vi "Begin.vi"() -> (0 "error out":errorcluster)   [LabVIEW 2013]
doc: "Called before other user functions, this VI is expected to open initial I/O refnums, load in file data, and do all program initialization. Notice that the <B>error out</B> terminal is simply used for data flow. Wiring it to other structures or subVIs ensures that this VI runs first."
uses:
  <vilib>/Rock Robotics/WPI/SafetyOutput/WPI_SafetyOutputConfigMenu.ctl
  <vilib>/Rock Robotics/WPI/DriverStation/WPI_DriverStationRobotMode2.ctl
  <vilib>/Rock Robotics/WPI/Joystick/WPI_JoystickDeviceEnum.ctl
  <vilib>/Rock Robotics/SystemInterfaces/DIO/FPGA_DIOPWMChannel.ctl
  <vilib>/Rock Robotics/SystemInterfaces/DIO/FPGA_DIORelayChannel.ctl
  <vilib>/Rock Robotics/WPI/Solenoid/WPI_SolenoidChannel.ctl
  <vilib>/Rock Robotics/SystemInterfaces/DIO/FPGA_DIOChannel.ctl
  <vilib>/Rock Robotics/SystemInterfaces/Typedef/FPGA_TypedefSolenoidModule.ctl
  <vilib>/Rock Robotics/WPI/Solenoid/WPI_SolenoidValue.ctl
  <vilib>/Rock Robotics/SystemInterfaces/Typedef/FPGA_TypedefAnalogModule.ctl
  <vilib>/Rock Robotics/SystemInterfaces/AI/FPGA_AIChannel.ctl
  <vilib>/Rock Robotics/SystemInterfaces/Typedef/FPGA_TypedefDigitalModule.ctl
  Robot Global Data.vi
  <vilib>/Rock Robotics/WPI/RobotDrive/WPI_RobotDriveOpen4MotorWithJaguar.vi
  <vilib>/Rock Robotics/WPI/MotorControl/WPI_MotorControlOpen Jaguar.vi
  <vilib>/Rock Robotics/WPI/Solenoid/WPI_SolenoidOpenDouble.vi
  <vilib>/Rock Robotics/WPI/Solenoid/WPI_SolenoidSetEnum.vi
  <vilib>/Rock Robotics/WPI/MotorControl/WPI_MotorControlOpen Victor.vi
  <vilib>/Rock Robotics/WPI/Compressor/WPI_CompressorGetSetRefNum.vi
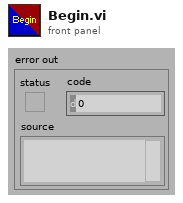
[diagram p1: front panel]
types:
  T1 = typedef "FPGA_TypedefDigitalModule.ctl" = enum16{"Digital Module 1", "Digital Module 2"}
  T2 = typedef "FPGA_DIORelayChannel.ctl" = enum8{"Relay 1", "Relay 2", "Relay 3", "Relay 4", "Relay 5", "Relay 6", "Relay 7", "Relay 8", "Invalid"}
  T3 = typedef "FPGA_AIChannel.ctl" = enum8{"AI 1", "AI 2", "AI 3", "AI 4", "AI 5", "AI 6", "AI 7", "AI 8", "Invalid"}
  T4 = typedef "FPGA_TypedefAnalogModule.ctl" = enum16{"Analog Module 1", "Analog Module 2"}
  T5 = typedef "WPI_SolenoidValue.ctl" = enum16{"Off", "On", "Forward", "Reverse"}
  T6 = typedef "WPI_SolenoidChannel.ctl" = enum8{"Solenoid 1", "Solenoid 2", "Solenoid 3", "Solenoid 4", "Solenoid 5", "Solenoid 6", "Solenoid 7", "Solenoid 8", "Invalid"}
  T7 = typedef "FPGA_TypedefSolenoidModule.ctl" = enum16{"Solenoid Module 1", "Solenoid Module 2"}
  T8 = typedef "FPGA_DIOPWMChannel.ctl" = enum8{"PWM 1", "PWM 2", "PWM 3", "PWM 4", "PWM 5", "PWM 6", "PWM 7", "PWM 8", "PWM 9", "PWM 10", "Invalid"}
  T9 = typedef "FPGA_DIOChannel.ctl" = enum8{"DIO 1", "DIO 2", "DIO 3", "DIO 4", "DIO 5", "DIO 6", "DIO 7", "DIO 8", "DIO 9", "DIO 10", "DIO 11", "DIO 12", "DIO 13", "DIO 14", "Invalid"}
  T10 = typedef "WPI_JoystickDeviceEnum.ctl" = enum16{"USB 1", "USB 2", "USB 3", "USB 4", "Kinect 1", "Kinect 2"}
  T11 = typedef "WPI_DriverStationRobotMode2.ctl" = enum16{"Autonomous Disabled", "Autonomous Enabled", "Teleop Disabled", "Teleop Enabled", "Timeout", "Finish", "Test Disabled", "Test Enabled"}
  T12 = typedef "WPI_SafetyOutputConfigMenu.ctl" = enum16{"Enable", "Disable"}
  T13 = typedef "WPI_MotorControlDeviceRef.ctl" = cluster{"DeviceStatus":errorcluster, "Type":enum16{"PWM", "CAN"}, "PWM":cluster{"Digital Module":T1, "PWM Channel":T8, "DeadBand":T14}, "CAN":cluster{"Device Number":u8, "Control Mode":T15, "Semaphore":T16, "Max Vout":dbl}, "Invert":bool, "TransformRef":T17, "InvTransformRef":T17}
  T14 = typedef "WPI_PWMDeadband.ctl" = cluster{"Name":string, "maxPositivePwm":i32, "minPositivePwm":i32, "centerPwm":i32, "maxNegativePwm":i32, "minNegativePwm":i32, "angularRange":u16}
  T15 = typedef "WPI_CANJaguar_ControlMode.ctl" = enum8{"Percent VBus", "Current", "Speed", "Position", "Voltage"}
  T16 = typedef "Semaphore RefNum" = refnum<k1>
  T17 = typedef "WPI_PWMTransform_ConPane.ctl" = refnum<vi>
  T18 = typedef "WPI_JoystickDevRef.ctl" = cluster{"Device":T10}
  T19 = typedef "WPI_RobotDriveDevRef.ctl" = cluster{"DevStatus":errorcluster, "Motors[]":T13[], "Square Inputs":bool, "Max Output":dbl, "Isochronous":bool}
  T20 = typedef "WPI_SolenoidDevRef.ctl" = cluster{"DevStatus":errorcluster, "Solenoid Module":T7, "Forward Solenoid Channel":T6, "Reverse Solenoid Channel":T6}
  T21 = typedef "WPI_RelayDevRef.ctl" = cluster{"DevStatus":errorcluster, "Relay Channel":T2, "Digital Module":T1, "Relay Direction":T22}
  T22 = typedef "WPI_RelayDirection.ctl" = enum16{"Both directions", "Forward only", "Reverse only"}
  T23 = typedef "WPI_CompressorDevRef.ctl" = cluster{"DevStatus":errorcluster, "DigitalInputDevRef":T24, "RelayDevRef":T21}
  T24 = typedef "WPI_DigitalInputDevRef.ctl" = cluster{"DevStatus":errorcluster, "DIO Channel":T9, "Digital Module":T1}
  T25 = typedef "WPI_AnalogChannelDevRef.ctl" = cluster{"DevStatus":errorcluster, "Analog Module":T4, "Analog Channel":T3}
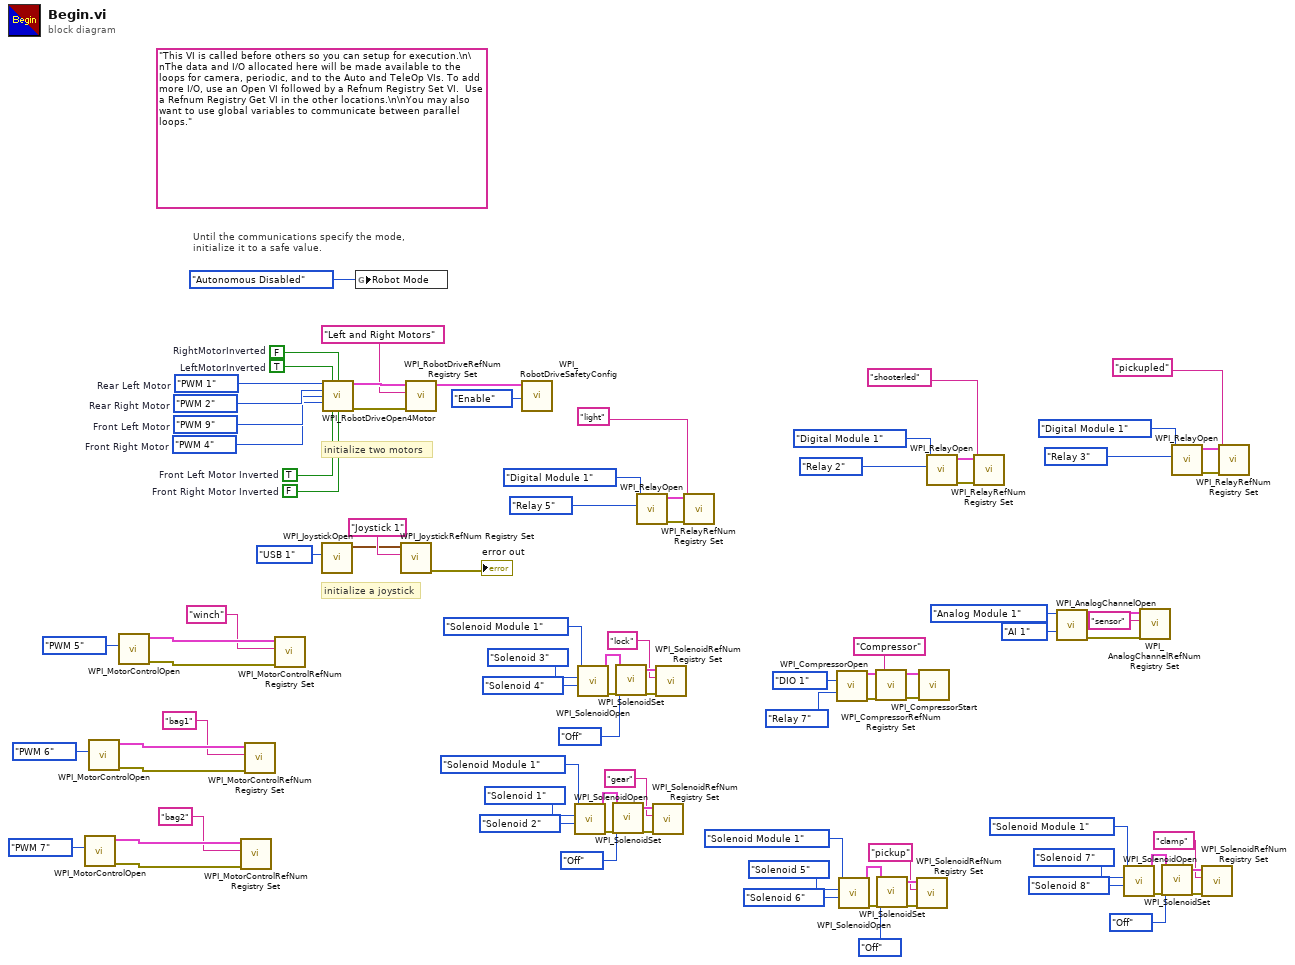
[diagram p0: block diagram]
diagram:
  w76 = FALSE  # Front Right Motor Inverted
  w77 = TRUE  # Front Left Motor Inverted
  w78 = FPGA_DIOPWMChannel."PWM 4"  # Front Right Motor
  w79 = FPGA_DIOPWMChannel."PWM 9"  # Front Left Motor
  w80 = FPGA_DIOPWMChannel."PWM 2"  # Rear Right Motor
  w81 = FPGA_DIOPWMChannel."PWM 1"  # Rear Left Motor
  (unwired) "This VI is called before others so you can setup for execution.\n\nThe data and I/O allocated here will be made available to the loops for camera, periodic, and to the Auto and TeleOp VIs. To add more I/O, use an Open VI followed by a Refnum Registry Set VI.  Use a Refnum Registry Get VI in the other locations.\n\nYou may also want to use global variables to communicate between parallel loops."
  w92 = TRUE  # LeftMotorInverted
  w93 = FALSE  # RightMotorInverted
  # "initialize a joystick"
  # "Until the communications specify the mode,\ninitialize it to a safe value."
  # "initialize two motors"
  n1 = call-poly <vilib>:"WPI_MotorControlOpen.vi"("PWM Channel"=FPGA_DIOPWMChannel."PWM 7") -> ("error out"=w32:errorcluster, "MotorControlDeviceRef"=w31:T13)  [unwired: 9 in]
  n2 = call-poly <vilib>:"WPI_MotorControlOpen.vi"("PWM Channel"=FPGA_DIOPWMChannel."PWM 6") -> ("error out"=w43:errorcluster, "MotorControlDeviceRef"=w42:T13)  [unwired: 9 in]
  n3 = call-poly <vilib>:"WPI_MotorControlOpen.vi"("PWM Channel"=FPGA_DIOPWMChannel."PWM 5") -> ("error out"=w69:errorcluster, "MotorControlDeviceRef"=w68:T13)  [unwired: 9 in]
  n4 = call <vilib>:"WPI_MotorControlRefNum Registry Set.vi"("error in (no error)"=w32, "refnum name"="bag2", "MotorControlDevRef"=w31) -> ()  [unwired: 7 in, 2 out]
  n5 = call <vilib>:"WPI_MotorControlRefNum Registry Set.vi"("error in (no error)"=w43, "refnum name"="bag1", "MotorControlDevRef"=w42) -> ()  [unwired: 7 in, 2 out]
  n6 = call <vilib>:"WPI_MotorControlRefNum Registry Set.vi"("error in (no error)"=w69, "refnum name"="winch", "MotorControlDevRef"=w68) -> ()  [unwired: 7 in, 2 out]
  n7 = call <vilib>:"WPI_JoystickOpen.vi"("JoystickDevice"=WPI_JoystickDeviceEnum."USB 1") -> ("JoystickDevRef"=w84:T18)  [unwired: 10 in]
  n8 = call-poly <vilib>:"WPI_RobotDriveOpen4Motor.vi"("Rear Left Motor"=w81, "Rear Left Motor Inverted"=w92, "Rear Right Motor Inverted"=w93, "Rear Right Motor"=w80, "Front Left Motor"=w79, "Front Right Motor"=w78, "Front Left Motor Inverted"=w77, "Front Right Motor Inverted"=w76) -> ("RobotDriveDevRef"=w91:T19, "error out"=w89:errorcluster)  [unwired: 6 in]
  n9 = global write "Robot Global Data.vi" "Robot Mode"(WPI_DriverStationRobotMode2."Autonomous Disabled" ("Robot Mode")) -> ()
  n10 = call <vilib>:"WPI_JoystickRefNum Registry Set.vi"("refnum name"="Joystick 1", "JoystickDevRef"=w84) -> ("error out"=→"error out":errorcluster)  [unwired: 8 in, 1 out]
  n11 = call <vilib>:"WPI_RobotDriveRefNum Registry Set.vi"("error in (no error)"=w89, "refnum name"="Left and Right Motors", "RobotDriveDevRef"=w91) -> ("RobotDriveDevRef"=w88:T19)  [unwired: 8 out]
  n12 = call <vilib>:"WPI_RobotDriveSafetyConfig.vi"("mode"=WPI_SafetyOutputConfigMenu."Enable", "RobotDriveDevRef"=w88) -> ()  [unwired: 8 in, 2 out]
  n13 = call-poly <vilib>:"WPI_SolenoidOpen.vi"("Reverse Solenoid Channel"=WPI_SolenoidChannel."Solenoid 2", "Forward Solenoid Channel"=WPI_SolenoidChannel."Solenoid 1" ("Solenoid Channel"), "Solenoid Module (Module 1)"=FPGA_TypedefSolenoidModule."Solenoid Module 1") -> ("error out"=w54:errorcluster, "SolenoidDevRef"=w53:T20)  [unwired: 7 in]
  n14 = call-poly <vilib>:"WPI_SolenoidOpen.vi"("Reverse Solenoid Channel"=WPI_SolenoidChannel."Solenoid 4", "Forward Solenoid Channel"=WPI_SolenoidChannel."Solenoid 3" ("Solenoid Channel"), "Solenoid Module (Module 1)"=FPGA_TypedefSolenoidModule."Solenoid Module 1") -> ("error out"=w63:errorcluster, "SolenoidDevRef"=w62:T20)  [unwired: 7 in]
  n15 = call-poly <vilib>:"WPI_SolenoidSet.vi"("error in (no error)"=w54, "Value"=WPI_SolenoidValue."Off", "SolenoidDevRef"=w53) -> ("error out"=w51:errorcluster, "SolenoidDevRef"=w52:T20)  [unwired: 7 in]
  n16 = call-poly <vilib>:"WPI_SolenoidSet.vi"("error in (no error)"=w63, "Value"=WPI_SolenoidValue."Off", "SolenoidDevRef"=w62) -> ("error out"=w60:errorcluster, "SolenoidDevRef"=w61:T20)  [unwired: 7 in]
  n17 = call <vilib>:"WPI_RelayOpen.vi"("Relay Channel"=FPGA_DIORelayChannel."Relay 5", "Digital Module (Module 1)"=FPGA_TypedefDigitalModule."Digital Module 1") -> ("error out"=w5:errorcluster, "RelayDevRef"=w4:T21)  [unwired: 8 in]
  n18 = call <vilib>:"WPI_SolenoidRefNum Registry Set.vi"("error in (no error)"=w51, "refnum name"="gear", "SolenoidDevRef"=w52) -> ()  [unwired: 7 in, 2 out]
  n19 = call <vilib>:"WPI_SolenoidRefNum Registry Set.vi"("error in (no error)"=w60, "refnum name"="lock", "SolenoidDevRef"=w61) -> ()  [unwired: 7 in, 2 out]
  n20 = call <vilib>:"WPI_RelayRefNum Registry Set.vi"("error in (no error)"=w5, "refnum name"="light", "RelayDevRef"=w4) -> ()  [unwired: 7 in, 2 out]
  n21 = call <vilib>:"WPI_CompressorOpen.vi"("Pressure Switch DIO Channel"=FPGA_DIOChannel."DIO 1", "Relay Channel"=FPGA_DIORelayChannel."Relay 7") -> ("CompressorDevRef"=w38:T23, "error out"=w39:errorcluster)  [unwired: 12 in]
  n22 = call-poly <vilib>:"WPI_SolenoidOpen.vi"("Reverse Solenoid Channel"=WPI_SolenoidChannel."Solenoid 6", "Forward Solenoid Channel"=WPI_SolenoidChannel."Solenoid 5" ("Solenoid Channel"), "Solenoid Module (Module 1)"=FPGA_TypedefSolenoidModule."Solenoid Module 1") -> ("error out"=w25:errorcluster, "SolenoidDevRef"=w24:T20)  [unwired: 7 in]
  n23 = call <vilib>:"WPI_CompressorRefNum Registry Set.vi"("error in (no error)"=w39, "refnum name"="Compressor", "CompressorDevRef"=w38) -> ("error out"=w37:errorcluster, "CompressorDevRef"=w36:T23)  [unwired: 7 in]
  n24 = call-poly <vilib>:"WPI_SolenoidSet.vi"("error in (no error)"=w25, "Value"=WPI_SolenoidValue."Off", "SolenoidDevRef"=w24) -> ("error out"=w22:errorcluster, "SolenoidDevRef"=w23:T20)  [unwired: 7 in]
  n25 = call <vilib>:"WPI_SolenoidRefNum Registry Set.vi"("error in (no error)"=w22, "refnum name"="pickup", "SolenoidDevRef"=w23) -> ()  [unwired: 7 in, 2 out]
  n26 = call <vilib>:"WPI_CompressorStart.vi"("error in (no error)"=w37, "CompressorDevRef"=w36) -> ()  [unwired: 8 in, 2 out]
  n27 = call <vilib>:"WPI_RelayOpen.vi"("Relay Channel"=FPGA_DIORelayChannel."Relay 2", "Digital Module (Module 1)"=FPGA_TypedefDigitalModule."Digital Module 1") -> ("error out"=w75:errorcluster, "RelayDevRef"=w74:T21)  [unwired: 8 in]
  n28 = call <vilib>:"WPI_RelayRefNum Registry Set.vi"("error in (no error)"=w75, "refnum name"="shooterled", "RelayDevRef"=w74) -> ()  [unwired: 7 in, 2 out]
  n29 = call <vilib>:"WPI_AnalogChannelOpen.vi"("Analog Channel"=FPGA_AIChannel."AI 1", "Analog Module (Module 1)"=FPGA_TypedefAnalogModule."Analog Module 1") -> ("error out"=w9:errorcluster, "AIDeviceRef"=w10:T25)  [unwired: 8 in]
  n30 = call-poly <vilib>:"WPI_SolenoidOpen.vi"("Reverse Solenoid Channel"=WPI_SolenoidChannel."Solenoid 8", "Forward Solenoid Channel"=WPI_SolenoidChannel."Solenoid 7" ("Solenoid Channel"), "Solenoid Module (Module 1)"=FPGA_TypedefSolenoidModule."Solenoid Module 1") -> ("error out"=w16:errorcluster, "SolenoidDevRef"=w15:T20)  [unwired: 7 in]
  n31 = call <vilib>:"WPI_AnalogChannelRefNum Registry Set.vi"("error in (no error)"=w9, "refnum name"="sensor", "AIDeviceRef"=w10) -> ()  [unwired: 7 in, 2 out]
  n32 = call-poly <vilib>:"WPI_SolenoidSet.vi"("error in (no error)"=w16, "Value"=WPI_SolenoidValue."Off", "SolenoidDevRef"=w15) -> ("error out"=w13:errorcluster, "SolenoidDevRef"=w14:T20)  [unwired: 7 in]
  n33 = call <vilib>:"WPI_RelayOpen.vi"("Relay Channel"=FPGA_DIORelayChannel."Relay 3", "Digital Module (Module 1)"=FPGA_TypedefDigitalModule."Digital Module 1") -> ("error out"=w48:errorcluster, "RelayDevRef"=w47:T21)  [unwired: 8 in]
  n34 = call <vilib>:"WPI_SolenoidRefNum Registry Set.vi"("error in (no error)"=w13, "refnum name"="clamp", "SolenoidDevRef"=w14) -> ()  [unwired: 7 in, 2 out]
  n35 = call <vilib>:"WPI_RelayRefNum Registry Set.vi"("error in (no error)"=w48, "refnum name"="pickupled", "RelayDevRef"=w47) -> ()  [unwired: 7 in, 2 out]
